vi "PathPlanner_PathFinder_ClearClosed.vi"(8 "error in (no error)":errorcluster) -> (0 "error out":errorcluster)   [LabVIEW 2019]
uses:
  PathPlannerLib24/TypeDef/PathPlannerFinderGridPosition.ctl
  PathPlannerLib24/VI/PathPlanner_PathFinder_Globals.vi
  PathPlannerLib24/PathPlanner24.lvlib
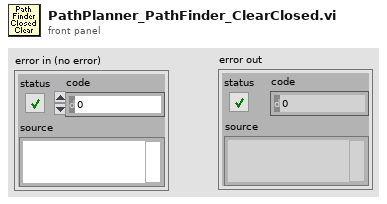
[diagram p1: front panel]
types:
  T1 = typedef "PathPlanner24.lvlib/PathPlannerFinderGridPosition.ctl" = cluster{"X":i32, "Y":i32}
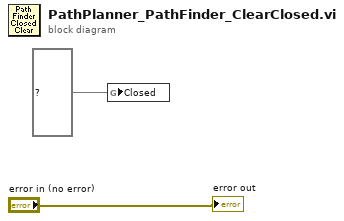
[diagram p0: block diagram]
diagram:
  n1 = global write "PathPlanner_PathFinder_Globals.vi" "Closed"(set{T1} {} ("Closed")) -> ()
  "error out" <- "error in (no error)"
